vi "Moving Average system.vi"(1 "M2":dbl=3.0, 2 "M1":dbl=2.0, 3 "Input Signal":dbl[](array[numeric])=[1.0, 2.0, 3.0, 2.0, 1.0, 2.0, 7.0, 2.0, 1.0, 3.0, 4.0, -16.0, 2.0, 3.0, -2.0, 5.0, 6.0, 1.0, 20.0, 0.0, 5.0, 2.0, 5.0, -2.0, 1.0, 3.0, -19.0, 2.0, 0.0, 0.0]) -> (0 "Moving Average Output":dbl[](array[numeric])=[1.3333333333333333, 1.5, 1.8333333333333333, 2.8333333333333335, 2.8333333333333335, 2.5, 2.6666666666666665, 3.1666666666666665, 0.16666666666666666, -0.6666666666666666, -0.5, -1.0, -0.6666666666666666, -0.3333333333333333, 2.5, 5.5, 5.0, 6.166666666666667, 5.666666666666667, 5.5, 5.0, 1.8333333333333333, 2.3333333333333335, -1.6666666666666667, -1.6666666666666667, -2.5, -2.1666666666666665, -2.3333333333333335, -2.8333333333333335, 0.3333333333333333])   [LabVIEW 2009]
panel:
  # "Moving Average System"
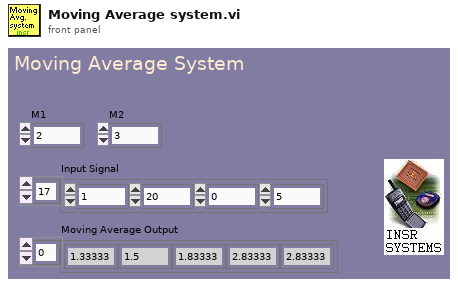
[diagram p1: front panel]
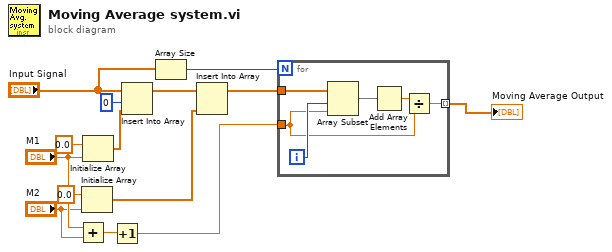
[diagram p0: block diagram]
diagram:
  n1 = Add(x="M1", y="M2") -> (x+y=w5:dbl)
  n2 = Initialize Array(0.0, "M2") -> (w9:dbl[])
  n3 = Initialize Array(0.0, "M1") -> (w13:dbl[])
  n4 = Increment(x=w5) -> (x+1=w3:dbl)
  n5 = Insert Into Array(array="Input Signal", index=0, new element=w13) -> (w11:dbl[])
  n6 = Array Size(array="Input Signal") -> (size(s)=w8:i32)
  n7 = Insert Into Array(array=w11, new element=w9) -> (w4:dbl[])  [unwired: 1 in]
  n8 = for {
    N: w8 -> [_]
    tunnel: w3 -> [w17]
    tunnel: w4 -> [w16]
    tunnel: [w18] -> w2 mode=indexing
    i -> [w20]
    n9 = Array Subset(array=w16, index=w20, length=w17) -> (w15:dbl[])
    n10 = Add Array Elements(numeric array=w15) -> (sum=w19:dbl)
    n11 = Divide(x=w19, y=w17) -> (x/y=w18:dbl)
  }
  "Moving Average Output" <- w2
